vi "Speed of VIight FPGA.vi"() -> ()   [LabVIEW 2026]
uses:
  <vilib>/rvi/Emulation/niFpgaGetClockAttributes.vi
  <vilib>/rvi/Emulation/niFpgaSctlEmulationGetInTimedLoop.vi
  <vilib>/rvi/Emulation/niFpgaEmulationReportErrorSimple.vi
  <vilib>/rvi/Emulation/niFpgaCriticalErrorInLSC.vi
  <vilib>/rvi/Emulation/niFpgaProcessEmulError.vi
  <vilib>/rvi/eio/common/nirviEmuTemplateMethod_errors.vi
  <vilib>/eio/EIONode/EIONode.xnode
panel:
  out "Player 2 Output 5":bool[](array[boolean])
  out "Player 1 Output 5":bool[](array[boolean])
  out "Initial 6 Random Numbers":u8[](array[numeric])
  out "Player 2 Bonus":u8
  out "Player 1 Bonus":u8
  in  "Max Bonus":u8=5
  in  "Bonus Threshold":u64=3000
  out "Intial Random Arrays":u8[](array[numeric])
  out "Player2 Input":bool[](array[boolean])
  out "Player1 Input":bool[](array[boolean])
  out "Player 2 Output 4":bool[](array[boolean])
  out "Player 2 Output 3":bool[](array[boolean])
  out "Player 2 Output 2":bool[](array[boolean])
  out "Player 2 Output 1":bool[](array[boolean])
  out "Player 1 Output 4":bool[](array[boolean])
  out "Player 1 Output 3":bool[](array[boolean])
  out "Player 1 Output 2":bool[](array[boolean])
  out "Player 2 Score":u32
  out "Player 2 Timer":u64
  out "Player 1 Score":u32
  out "Player 1 Timer":u64
  out "Main Loop":i32
  out "Closing Loop":i32
  out "Element to change 2":i32
  out "Element to change":i32
  out "Measured Main Loop Ticks":u32
  in  "Main Loop Timer":u32=1 caption="Main Loop Timer (uSec)"
  out "Player2 Output Number":u32
  out "Player1 Output Number":u32
  out "Initialized Array 2":bool[](array[boolean])
  out "Initialized Array 1":bool[](array[boolean])
  out "Random Number":u8
  in  "Random Number Max":u8=20
  out "Idle Loop":i32
  out "Current State":i16
  out "Blue2":bool
  out "Green3":bool
  out "Green2":bool
  out "Blue1":bool
  out "Green1":bool
  out "Player 1 Output":bool[](array[boolean])
  in  "Game Length (s)":u32=45
  in  "Stop Closing Loop":bool
  in  "Stop Main Loop":bool
  in  "Stop Idle":bool
  in  "Global Stop":bool
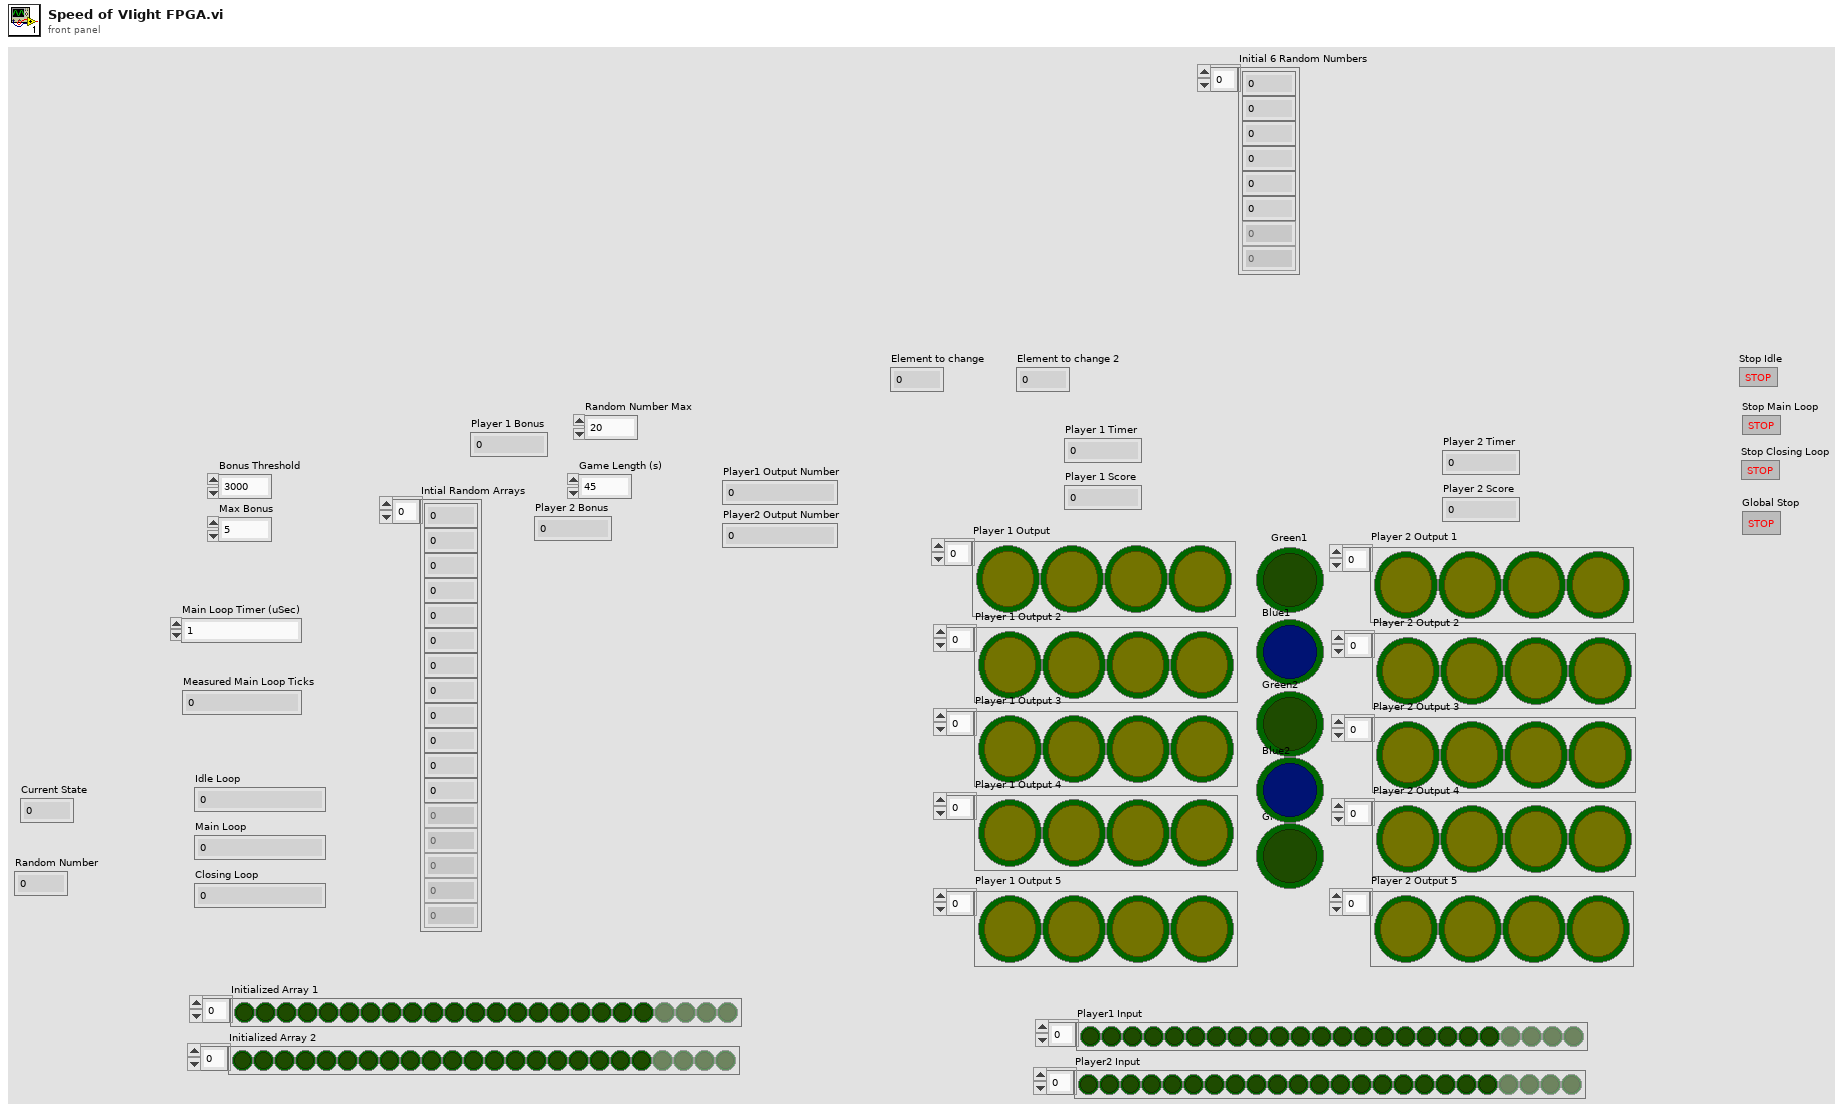
[diagram p1: front panel]
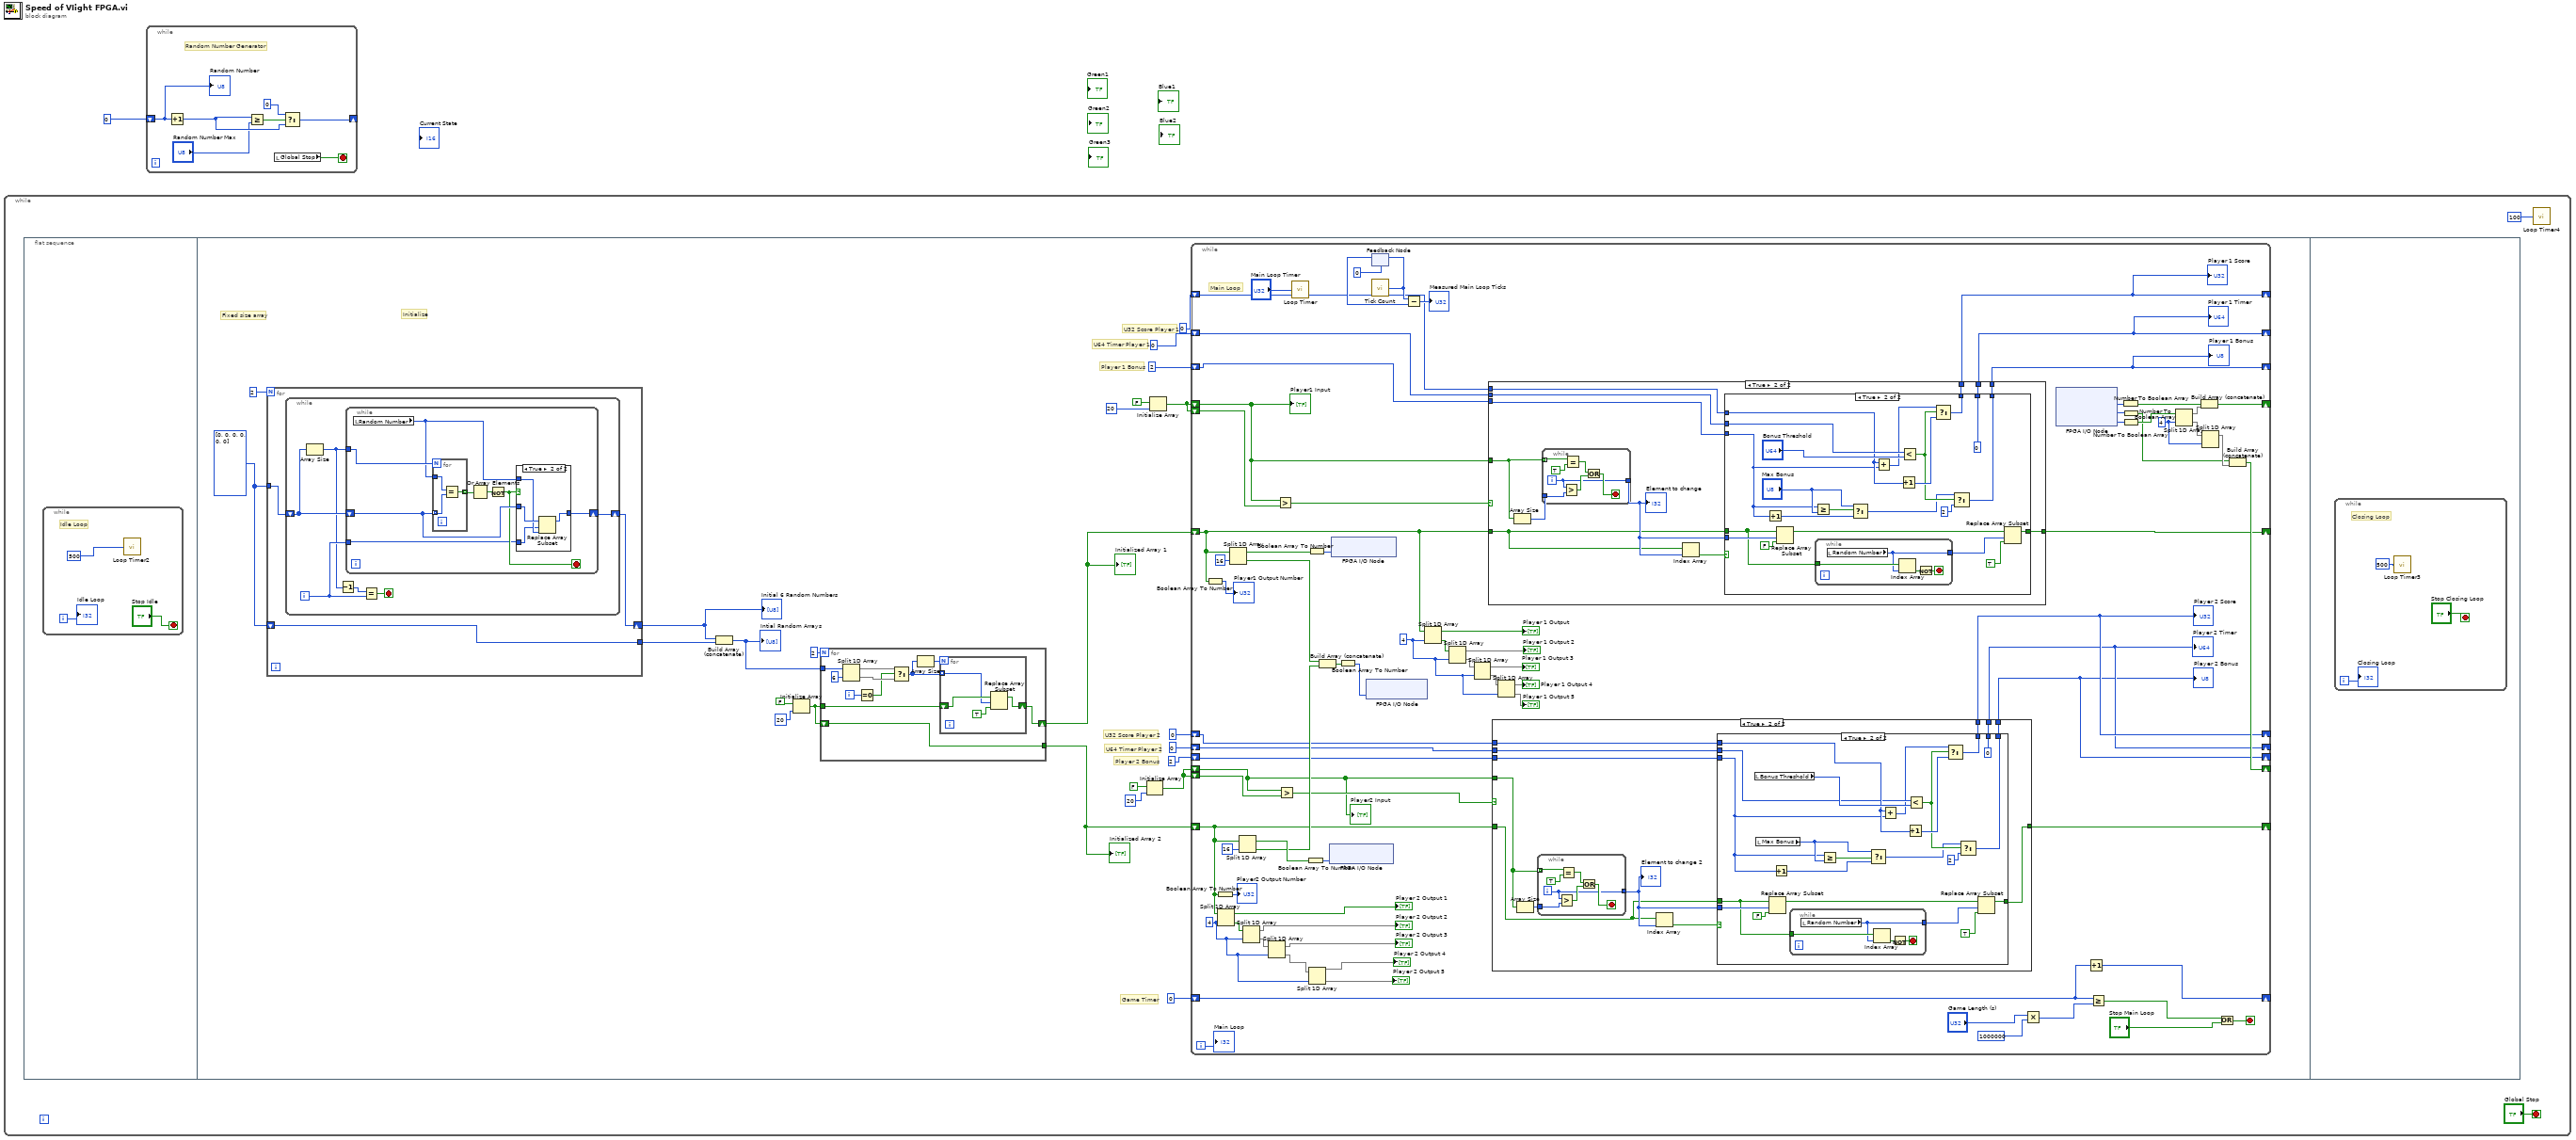
[diagram p0: block diagram]
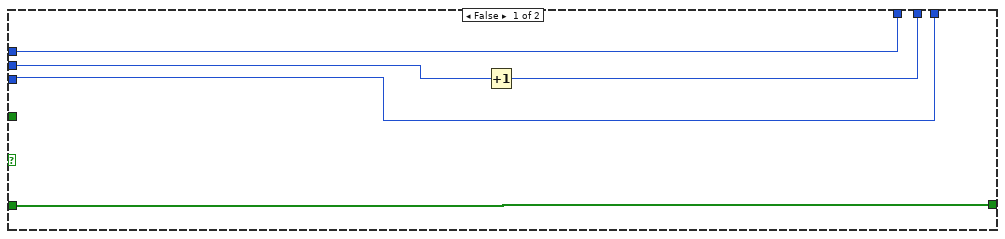
[diagram p3: hidden frame]
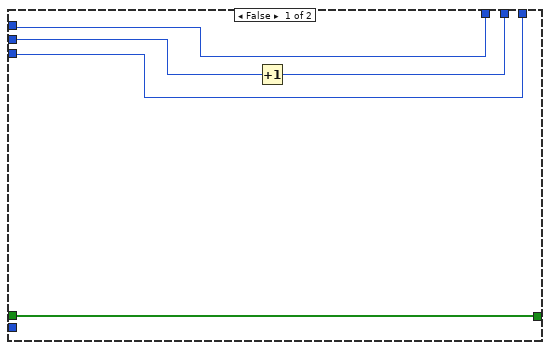
[diagram p4: hidden frame]
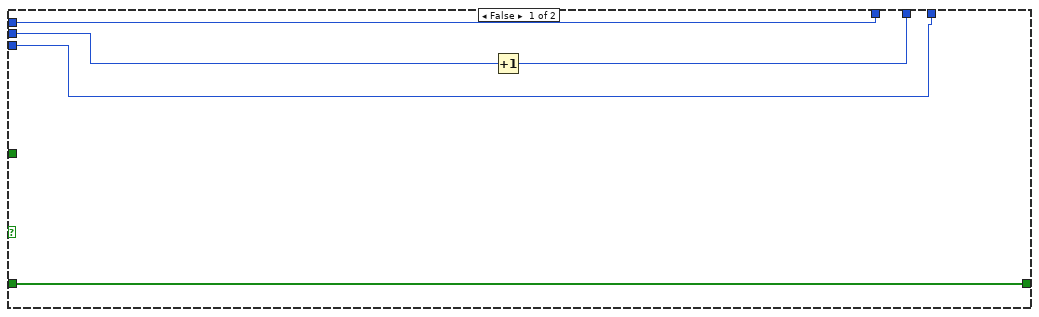
[diagram p5: hidden frame]
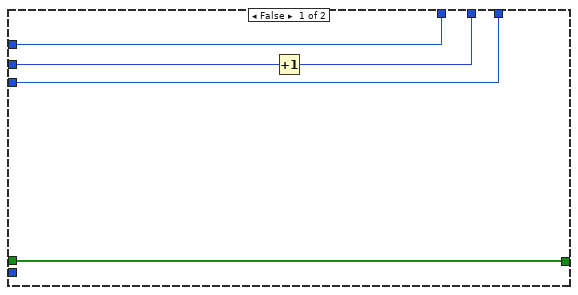
[diagram p6: hidden frame]
diagram:
  n1 = while {
    stop <- "Global Stop" stop-if-true
    n2 = flat-sequence {
      frame #0 {
        n3 = while {
          i -> [w5]
          stop <- "Stop Idle" stop-if-true
          # "Idle Loop"
          n4 = call "Loop Timer2"("Count(mSec)"=u32 500 ("millisecond multiple")) -> ()  [unwired: 1 out]
          "Idle Loop" <- w5
        }
      }
      frame #1 {
        w12 = u8[] [0, 0, 0, 0, 0, 0] ("Initial Random Numbers")
        # "Player 2 Bonus"
        # "Player 1 Bonus"
        # "Initialize"
        # "Fixed size array"
        # "Game Timer"
        # "U32 Score Player 2"
        # "U32 Score Player 1"
        # "U64 Timer Player 2"
        # "U64 Timer Player 1"
        n5 = for {
          N: 2 -> [_]
          tunnel: w12 -> [w48]
          shift-right: [w47] -> w11
          shift-left: w12 -> [w46]
          tunnel: [w46] -> w10
          n6 = while {
            shift-right: [w51] -> w47
            shift-left: w48 -> [w52]
            i -> [w54]
            stop <- w53 stop-if-true
            n7 = Array Size(array=w52) -> (size(s)=w49:i32)
            n8 = Decrement(x=w49) -> (x-1=w50:i32)
            n9 = while {
              tunnel: w54 -> [w56]
              shift-right: [w57] -> w51
              shift-left: w52 -> [w59]
              tunnel: w49 -> [w62]
              stop <- w58 stop-if-true
              n10 = local read "Random Number"() -> (w55:u8)
              n11 = for {
                N: w62 -> [_]
                tunnel: w59 -> [w69] mode=indexing
                tunnel: w55 -> [w70]
                tunnel: [w68] -> w61 mode=indexing
                n12 = Equal?(x=w70, y=w69) -> (x = y?=w68:bool)
              }
              n13 = Or Array Elements(Boolean array=w61) -> (logical OR=w60:bool)
              n14 = Not(x=w60) -> (.not. x?=w58:bool)
              n15 = case shown="True" w58 {
                tunnel: w59 -> [w63 w67]
                tunnel: [w63 w66] -> w57
                tunnel: w55 -> [_ w65]
                tunnel: w56 -> [_ w64]
                frame False {
                }
                frame True {
                  n16 = Replace Array Subset(array=w67, new element=w65, index=w64) -> (w66:u8[])
                }
              }
            }
            n17 = Equal?(x=w50, y=w54) -> (x = y?=w53:bool)
          }
        }
        "Initial 6 Random Numbers" <- w11
        n18 = Build Array (concatenate)(w11, w10) -> (w9:u8[])
        "Intial Random Arrays" <- w9
        n19 = Initialize Array(FALSE ("Boolean"), 20 ("dimension size")) -> (w13:bool[])
        n20 = for {
          N: 2 -> [_]
          tunnel: w13 -> [w40]
          tunnel: w9 -> [w38]
          shift-right: [w41] -> w8
          shift-left: w13 -> [w31]
          tunnel: [w31] -> w7
          i -> [w34]
          n21 = Split 1D Array(array=w38, index=6) -> (first subarray=w35:u8[], second subarray=w36:u8[])
          n22 = Equal To 0?(x=w34) -> (x = 0?=w33:bool)
          n23 = Select(t=w35, s=w33, f=w36) -> (s? t:f=w32:u8[])
          n24 = Array Size(array=w32) -> (size(s)=w39:i32)
          n25 = for {
            N: w39 -> [_]
            tunnel: w32 -> [w42] mode=indexing
            shift-right: [w45] -> w41
            shift-left: w40 -> [w44]
            n26 = Replace Array Subset(array=w44, new element=TRUE ("new element/subarray"), index=w42) -> (w45:bool[])
          }
        }
        "Initialized Array 1" <- w8
        "Initialized Array 2" <- w7
        n27 = Initialize Array(FALSE ("Boolean"), 20 ("dimension size")) -> (w14:bool[])
        n28 = Initialize Array(FALSE ("Boolean"), 20 ("dimension size")) -> (w17:bool[])
        n29 = while {
          shift-right: [w88] -> _
          shift-left: u64 0 -> [w92]
          shift-right: [w82] -> _
          shift-left: u64 0 -> [w86]
          shift-right: [w90] -> _
          shift-left: u32 0 -> [w91]
          shift-right: [w83] -> _
          shift-left: u32 0 -> [w84]
          shift-right: [w146] -> _
          shift-left: u32 0 -> [w147]
          shift-right: [w116] -> _
          shift-left: w8 -> [w98]
          shift-right: [w113] -> _
          shift-left: w7 -> [w106]
          shift-right: [w121] -> _
          shift-left: w17 -> [w94]
          shift-right: [w120] -> _
          shift-left: w14 -> [w93]
          shift-left: w17 -> [w119]
          shift-left: w14 -> [w115]
          shift-right: [w87] -> _
          shift-left: u8 2 -> [w89]
          shift-right: [w81] -> _
          shift-left: u8 2 -> [w85]
          i -> [w108]
          stop <- w112 stop-if-true
          w71 = 4 ("index")
          w78 = 4 ("index")
          w127 = 4 ("index")
          # "Main Loop"
          n30 = Boolean Array To Number(Boolean array=w98) -> (number=→"Player1 Output Number":u32)
          n31 = Boolean Array To Number(Boolean array=w106) -> (number=→"Player2 Output Number":u32)
          n32 = Split 1D Array(array=w106, index=w78) -> (first subarray=→"Player 2 Output 1":bool[], second subarray=w104:bool[])
          n33 = Split 1D Array(array=w98, index=16) -> (first subarray=w117:bool[], second subarray=w137:bool[])
          n34 = Split 1D Array(array=w106, index=16) -> (first subarray=w140:bool[], second subarray=w136:bool[])
          n35 = Split 1D Array(array=w104, index=w78) -> (first subarray=→"Player 2 Output 2":bool[], second subarray=w102:bool[])
          n36 = Split 1D Array(array=w102, index=w78) -> (first subarray=→"Player 2 Output 3":bool[], second subarray=w76:bool[])
          n37 = Greater?(x=w94, y=w119) -> (0:w118:bool)
          n38 = Greater?(x=w93, y=w115) -> (0:w114:bool)
          n39 = call "Loop Timer"("Count(uSec)"="Main Loop Timer") -> ()  [unwired: 1 out]
          n40 = Boolean Array To Number(Boolean array=w140) -> (number=w139:u32)
          n41 = Boolean Array To Number(Boolean array=w117) -> (number=w142:u32)
          n42 = Split 1D Array(array=w76, index=w78) -> (first subarray=→"Player 2 Output 4":bool[], second subarray=→"Player 2 Output 5":bool[])
          n43 = Build Array (concatenate)(w137, w136) -> (w135:bool[])
          n44 = xnode "FPGA I/O Node"("Mod7/DO15:0"=w139) -> ()  [unwired: 1 in, 1 out]
          n45 = xnode "FPGA I/O Node"("Mod6/DO15:0"=w142) -> ()  [unwired: 1 in, 1 out]
          n46 = Boolean Array To Number(Boolean array=w135) -> (number=w134:u32)
          n47 = xnode "FPGA I/O Node"("Mod8/DO7:0"=w134) -> ()  [unwired: 1 in, 1 out]
          n48 = feedback #1(u32 0) -> (w124:u32)
          n49 = call "Tick Count"() -> ("Tick Count(Ticks)"=w123:u32)
          n50 = feedback-in #1(w123) -> ()
          n51 = Subtract(x=w123, y=w124) -> (x-y=→"Measured Main Loop Ticks":u32)
          n52 = Split 1D Array(array=w98, index=w71) -> (first subarray=→"Player 1 Output":bool[], second subarray=w100:bool[])
          n53 = Split 1D Array(array=w100, index=w71) -> (first subarray=→"Player 1 Output 2":bool[], second subarray=w99:bool[])
          n54 = Split 1D Array(array=w99, index=w71) -> (first subarray=→"Player 1 Output 3":bool[], second subarray=w74:bool[])
          n55 = case shown="True" w118 {
            tunnel: [w208 w220] -> w116
            tunnel: w94 -> [_ w217]
            tunnel: w98 -> [w208 w215]
            tunnel: w92 -> [w206 w211]
            tunnel: [w205 w213] -> w88
            tunnel: w91 -> [w207 w212]
            tunnel: [w207 w214] -> w90
            tunnel: w89 -> [w204 w210]
            tunnel: [w204 w209] -> w87
            frame False {
              n56 = Increment(x=w206) -> (x+1=w205:u64)
            }
            frame True {
              n57 = Array Size(array=w217) -> (size(s)=w216:i32)
              n58 = while {
                tunnel: w217 -> [w258] mode=indexing
                tunnel: w216 -> [w254]
                tunnel: [w252] -> w219
                i -> [w252]
                stop <- w255 stop-if-true
                n59 = Greater?(x=w252, y=w254) -> (0:w253:bool)
                n60 = Equal?(x=w258, y=TRUE ("element")) -> (x = y?=w256:bool)
                n61 = Or(x=w256, y=w253) -> (x .or. y?=w255:bool)
              }
              "Element to change" <- w219
              n62 = Index Array(array=w215, index=w219) -> (element=w218:bool)
              n63 = case shown="True" w218 {
                tunnel: w219 -> [_ w247]
                tunnel: [w225 w243] -> w220
                tunnel: w215 -> [w225 w241]
                tunnel: w212 -> [w224 w228]
                tunnel: w211 -> [w223 w239]
                tunnel: [w224 w237] -> w214
                tunnel: [w222 u64 0] -> w213
                tunnel: w210 -> [w221 w227]
                tunnel: [w221 w234] -> w209
                frame False {
                  n64 = Increment(x=w223) -> (x+1=w222:u64)
                }
                frame True {
                  n65 = Increment(x=w227) -> (x+1=w230:u8)
                  n66 = Replace Array Subset(array=w241, new element=FALSE ("new element/subarray"), index=w247) -> (w245:bool[])
                  n67 = Greater Or Equal?(x=w227, y="Max Bonus") -> (x >= y?=w232:bool)
                  n68 = while {
                    tunnel: [w248] -> w242
                    tunnel: w241 -> [w251]
                    stop <- w249 stop-if-true
                    n69 = local read "Random Number"() -> (w248:u8)
                    n70 = Index Array(array=w251, index=w248) -> (element=w250:bool)
                    n71 = Not(x=w250) -> (.not. x?=w249:bool)
                  }
                  n72 = Select(t="Max Bonus", s=w232, f=w230) -> (s? t:f=w229:u8)
                  n73 = Add(x=w228, y=w227) -> (x+y=w226:u32)
                  n74 = Increment(x=w228) -> (x+1=w238:u32)
                  n75 = Less?(x=w239, y="Bonus Threshold") -> (x < y?=w236:bool)
                  n76 = Select(t=w226, s=w236, f=w238) -> (s? t:f=w237:u32)
                  n77 = Select(t=w229, s=w236, f=u8 2) -> (s? t:f=w234:u8)
                  n78 = Replace Array Subset(array=w245, new element=TRUE ("new element/subarray"), index=w242) -> (w243:bool[])
                }
              }
            }
          }
          "Player 1 Timer" <- w88
          "Player 1 Score" <- w90
          "Player 1 Bonus" <- w87
          n79 = case shown="True" w114 {
            tunnel: [w153 w161] -> w113
            tunnel: w93 -> [_ w163]
            tunnel: w106 -> [w153 w160]
            tunnel: w86 -> [w151 w158]
            tunnel: w85 -> [w149 w157]
            tunnel: w84 -> [w152 w159]
            tunnel: [w152 w155] -> w83
            tunnel: [w150 w156] -> w82
            tunnel: [w149 w154] -> w81
            frame False {
              n80 = Increment(x=w151) -> (x+1=w150:u64)
            }
            frame True {
              n81 = Array Size(array=w163) -> (size(s)=w162:i32)
              n82 = while {
                tunnel: w163 -> [w203] mode=indexing
                tunnel: w162 -> [w199]
                tunnel: [w197] -> w165
                i -> [w197]
                stop <- w200 stop-if-true
                n83 = Greater?(x=w197, y=w199) -> (0:w198:bool)
                n84 = Equal?(x=w203, y=TRUE ("element")) -> (x = y?=w201:bool)
                n85 = Or(x=w201, y=w198) -> (x .or. y?=w200:bool)
              }
              "Element to change 2" <- w165
              n86 = Index Array(array=w160, index=w165) -> (element=w164:bool)
              n87 = case shown="True" w164 {
                tunnel: w165 -> [_ w192]
                tunnel: [w170 w188] -> w161
                tunnel: w160 -> [w170 w186]
                tunnel: w159 -> [w166 w178]
                tunnel: w158 -> [w169 w173]
                tunnel: w157 -> [w167 w171]
                tunnel: [w168 u64 0] -> w156
                tunnel: [w167 w176] -> w154
                tunnel: [w166 w175] -> w155
                frame False {
                  n88 = Increment(x=w169) -> (x+1=w168:u64)
                }
                frame True {
                  n89 = local read "Bonus Threshold"() -> (w180:u64)
                  n90 = local read "Max Bonus"() -> (w179:u8)
                  n91 = Replace Array Subset(array=w186, new element=FALSE ("new element/subarray"), index=w192) -> (w190:bool[])
                  n92 = Increment(x=w171) -> (x+1=w174:u8)
                  n93 = while {
                    tunnel: [w193] -> w187
                    tunnel: w186 -> [w196]
                    stop <- w194 stop-if-true
                    n94 = local read "Random Number"() -> (w193:u8)
                    n95 = Index Array(array=w196, index=w193) -> (element=w195:bool)
                    n96 = Not(x=w195) -> (.not. x?=w194:bool)
                  }
                  n97 = Greater Or Equal?(x=w171, y=w179) -> (x >= y?=w182:bool)
                  n98 = Select(t=w179, s=w182, f=w174) -> (s? t:f=w181:u8)
                  n99 = Add(x=w178, y=w171) -> (x+y=w172:u32)
                  n100 = Increment(x=w178) -> (x+1=w185:u32)
                  n101 = Less?(x=w173, y=w180) -> (x < y?=w184:bool)
                  n102 = Select(t=w172, s=w184, f=w185) -> (s? t:f=w175:u32)
                  n103 = Select(t=w181, s=w184, f=u8 2) -> (s? t:f=w176:u8)
                  n104 = Replace Array Subset(array=w190, new element=TRUE ("new element/subarray"), index=w187) -> (w188:bool[])
                }
              }
            }
          }
          "Player 2 Timer" <- w82
          "Player 2 Score" <- w83
          "Player 2 Bonus" <- w81
          n105 = Split 1D Array(array=w74, index=w71) -> (first subarray=→"Player 1 Output 4":bool[], second subarray=→"Player 1 Output 5":bool[])
          n106 = Multiply(x="Game Length (s)", y=u32 1000000) -> (x*y=w109:u32)
          n107 = xnode "FPGA I/O Node"() -> ("Mod6/DI15:0"=w133:u16, "Mod7/DI15:0"=w132:u16, "Mod8/DI15:0"=w131:u16)  [unwired: 3 in, 3 out]
          n108 = Increment(x=w147) -> (x+1=w146:u32)
          n109 = Greater Or Equal?(x=w147, y=w109) -> (x >= y?=w145:bool)
          n110 = Number To Boolean Array(number=w133) -> (Boolean array=w129:bool[])
          n111 = Number To Boolean Array(number=w132) -> (Boolean array=w79:bool[])
          n112 = Number To Boolean Array(number=w131) -> (Boolean array=w80:bool[])
          n113 = Split 1D Array(array=w80, index=w127) -> (first subarray=w128:bool[], second subarray=w126:bool[])
          n114 = Build Array (concatenate)(w129, w128) -> (w121:bool[])
          n115 = Split 1D Array(array=w126, index=w127) -> (first subarray=w125:bool[])  [unwired: 1 out]
          n116 = Or(x=w145, y="Stop Main Loop") -> (x .or. y?=w112:bool)
          n117 = Build Array (concatenate)(w79, w125) -> (w120:bool[])
          "Main Loop" <- w108
          "Player1 Input" <- w94
          "Player2 Input" <- w93
        }
      }
      frame #2 {
        n118 = while {
          i -> [w260]
          stop <- "Stop Closing Loop" stop-if-true
          # "Closing Loop"
          n119 = call "Loop Timer3"("Count(mSec)"=u32 500 ("millisecond multiple")) -> ()  [unwired: 1 out]
          "Closing Loop" <- w260
        }
      }
    }
    n120 = call "Loop Timer4"("Count(mSec)"=u32 100 ("millisecond multiple")) -> ()  [unwired: 1 out]
  }
  n121 = while {
    shift-right: [w266] -> _
    shift-left: u8 0 -> [w268]
    stop <- w262 stop-if-true
    # "Random Number Generator"
    n122 = Increment(x=w268) -> (x+1=w265:u8)
    n123 = Greater Or Equal?(x=w265, y="Random Number Max") -> (x >= y?=w264:bool)
    n124 = local read "Global Stop"() -> (w262:bool)
    n125 = Select(t=u8 0, s=w264, f=w265) -> (s? t:f=w266:u8)
    "Random Number" <- w268
  }
